vi "num-cmd-test.vi"() -> ()   [LabVIEW 2019]
uses:
  <vilib>/Rock Robotics/WPI/ThirdParty/JAS_Junk/TrajLib/VI/numCmd_Recv_Generic.vi
  <vilib>/Rock Robotics/WPI/ThirdParty/JAS_Junk/TrajLib/VI/numCmd_Send_Generic.vi
  <vilib>/Rock Robotics/WPI/ThirdParty/JAS_Junk/TrajLib/VI/numCmd_ObtainQueue.vi
  <vilib>/Rock Robotics/WPI/ThirdParty/JAS_Junk/TrajLib/VI/numCmd_Send_Internal.vi
  <vilib>/Rock Robotics/WPI/ThirdParty/JAS_Junk/TrajLib/Trajectory_Library.lvlib
  <vilib>/Rock Robotics/WPI/ThirdParty/JAS_Junk/TrajLib/TypeDef/CHASSIS_SPEEDS.ctl
panel:
  out "Chassis Speeds 2":T1 {"vOmega" format="%10.3f"; "vY" format="%10.3f"; "vX" format="%10.3f"}
  out "Changed 5":bool
  out "error out 10":errorcluster
  in  "Chassis Speeds":T1 {"vOmega" format="%10.3f"; "vY" format="%10.3f"; "vX" format="%10.3f"}
  out "error out 9":errorcluster
  out "error out 4":errorcluster
  out "Changed 4":bool
  out "One 3":dbl[](array[numeric])
  out "error out 8":errorcluster
  in  "Test 4":dbl[](array[numeric])
  out "Value 3":dbl
  out "Changed 3":bool
  out "One 2":dbl
  out "error out 7":errorcluster
  in  "Value 2":dbl
  out "error out":errorcluster
  in  "Test 3":dbl
  out "Changed 2":bool
  out "Changed 1":bool
  out "Two":dbl
  out "One":dbl
  out "error out 6":errorcluster
  out "error out 5":errorcluster
  out "error out 3":errorcluster
  out "error out 2":errorcluster
  in  "milliseconds to wait 2":u32=250
  in  "milliseconds to wait":u32=250
  in  "Test 2":dbl
  in  "Test 1":dbl
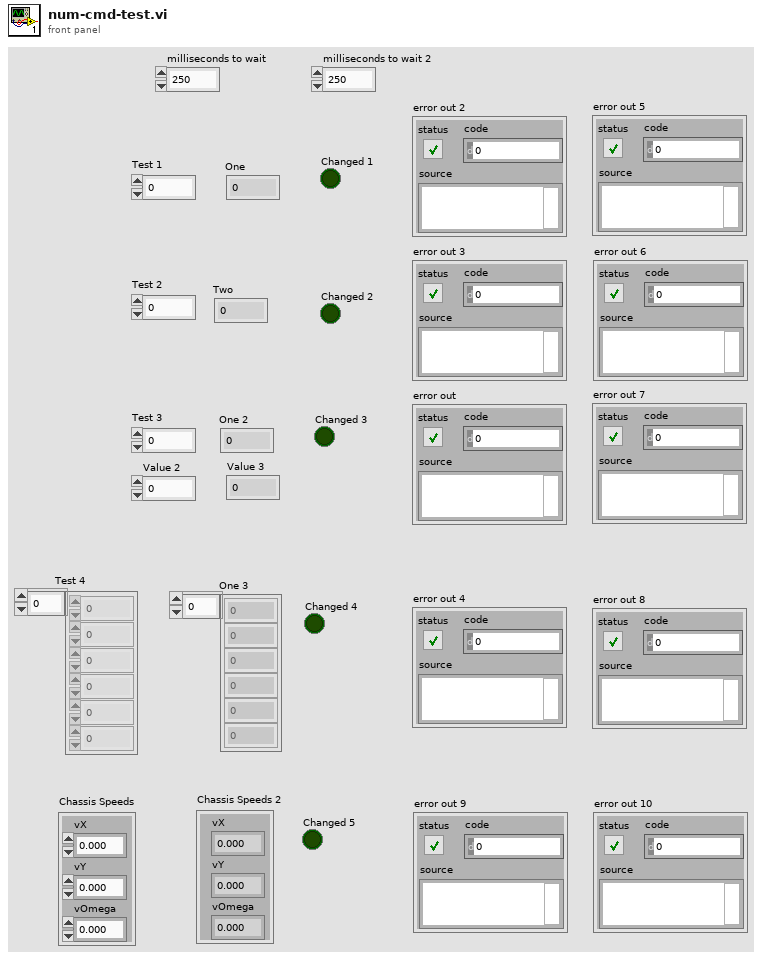
[diagram p1: front panel]
types:
  T1 = typedef "Trajectory_Library.lvlib/CHASSIS_SPEEDS.ctl" = cluster{"vX":dbl, "vY":dbl, "vOmega":dbl}
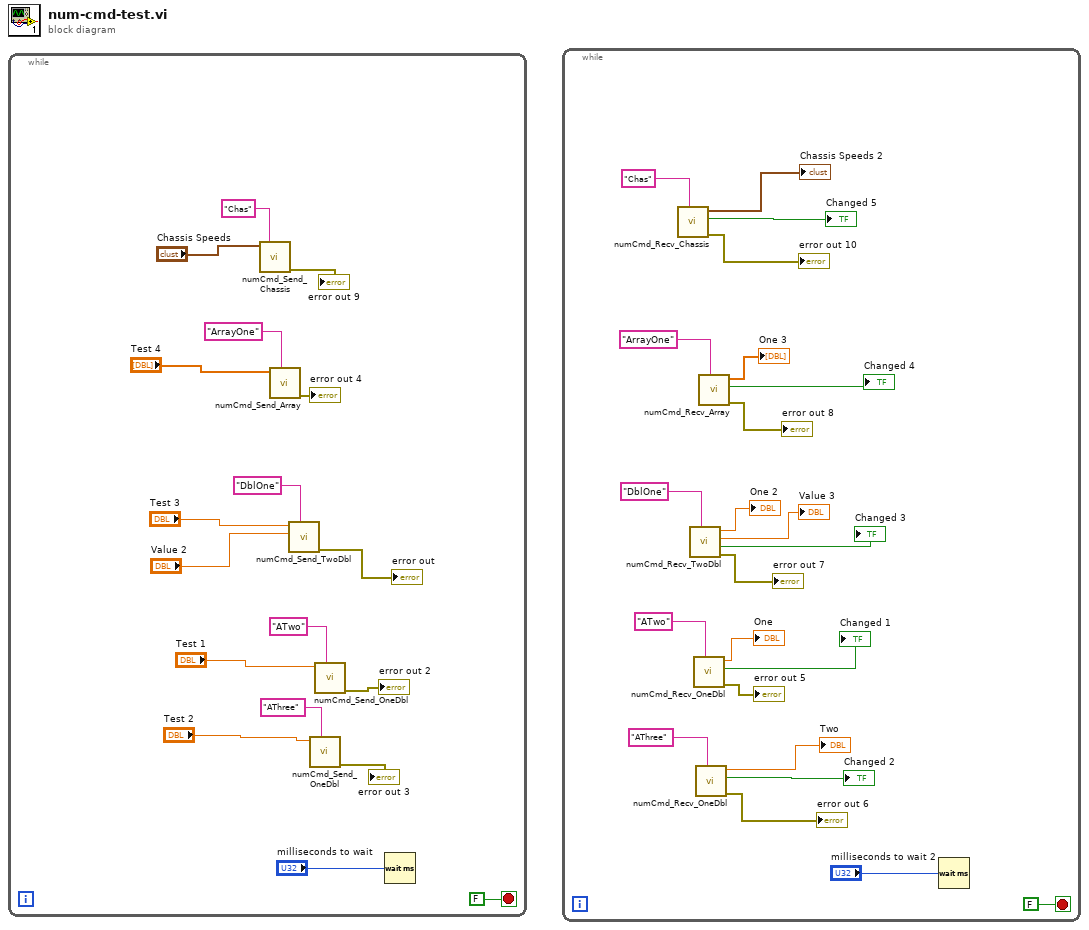
[diagram p0: block diagram]
diagram:
  n1 = while {
    stop <- FALSE stop-if-true
    n2 = call <vilib>:"numCmd_Send_Chassis.vi"("Command Name"="Chas", "Chassis Speeds"="Chassis Speeds") -> ("error out"=→"error out 9":errorcluster)  [unwired: 9 in]
    n3 = call <vilib>:"numCmd_Send_Array.vi"("Command Name"="ArrayOne", "Values"="Test 4") -> ("error out"=→"error out 4":errorcluster)  [unwired: 9 in]
    n4 = call <vilib>:"numCmd_Send_TwoDbl.vi"("Command Name"="DblOne", "Value 2"="Value 2", "Value 1"="Test 3") -> ("error out"=→"error out":errorcluster)  [unwired: 8 in]
    n5 = call <vilib>:"numCmd_Send_OneDbl.vi"("Command Name"="AThree", "Value"="Test 2") -> ("error out"=→"error out 3":errorcluster)  [unwired: 9 in]
    n6 = call <vilib>:"numCmd_Send_OneDbl.vi"("Command Name"="ATwo", "Value"="Test 1") -> ("error out"=→"error out 2":errorcluster)  [unwired: 9 in]
    n7 = Wait (ms)(milliseconds to wait="milliseconds to wait") -> ()  [unwired: 1 out]
  }
  n8 = while {
    stop <- FALSE stop-if-true
    n9 = call <vilib>:"numCmd_Recv_Chassis.vi"("Command Name"="Chas") -> ("error out"=→"error out 10":errorcluster, "Any Changed"=→"Changed 5":bool, "Chassis Speeds"=→"Chassis Speeds 2":T1)  [unwired: 8 in]
    n10 = call <vilib>:"numCmd_Recv_TwoDbl.vi"("Command Name"="DblOne") -> ("error out"=→"error out 7":errorcluster, "Any Changed"=→"Changed 3":bool, "Value 2"=→"Value 3":dbl, "Value 1"=→"One 2":dbl)  [unwired: 7 in]
    n11 = call <vilib>:"numCmd_Recv_OneDbl.vi"("Command Name"="ATwo") -> ("error out"=→"error out 5":errorcluster, "Changed"=→"Changed 1":bool, "Value"=→"One":dbl)  [unwired: 8 in]
    n12 = call <vilib>:"numCmd_Recv_OneDbl.vi"("Command Name"="AThree") -> ("error out"=→"error out 6":errorcluster, "Changed"=→"Changed 2":bool, "Value"=→"Two":dbl)  [unwired: 8 in]
    n13 = call <vilib>:"numCmd_Recv_Array.vi"("Command Name"="ArrayOne") -> ("error out"=→"error out 8":errorcluster, "Any Changed"=→"Changed 4":bool, "Values"=→"One 3":dbl[])  [unwired: 8 in]
    n14 = Wait (ms)(milliseconds to wait="milliseconds to wait 2") -> ()  [unwired: 1 out]
  }
